vi "Select Global Control.vi"(6 "Variant in":variant, 7 "Shift Pressed?":bool, 8 "error in (no error)":errorcluster, 10 "QD Combo Box Ref":refnum<vi>, 11 "QD Launch VI Ref":refnum<vi>) -> (0 "error out":errorcluster, 4 "Variant out":variant)   [LabVIEW 2017]
doc: "This plugin automatically changes the selected global's selected control. To use it, select the global you want to change, open quickdrop (Ctrl+Space), type the name of the control you want to select from the global, then use this plugin (by default, Ctrl+G).\n\nThe name is case sensitive. If the text in quickdrop does not match any of the controls in the global, or if no global is selected, this plugin does nothing.\n\nDefault Shortcut - [G]"
uses:
  <vilib>/ErrorRing/Error Ring.xnode
panel:
  in  "Undo Name":string="Quick Drop Keyboard Shortcut"
  # "Do not change the connector pane of this VI.\n\nSee the block diagram for directions on how to use this template."
  # "Specify the name of the Undo transaction"
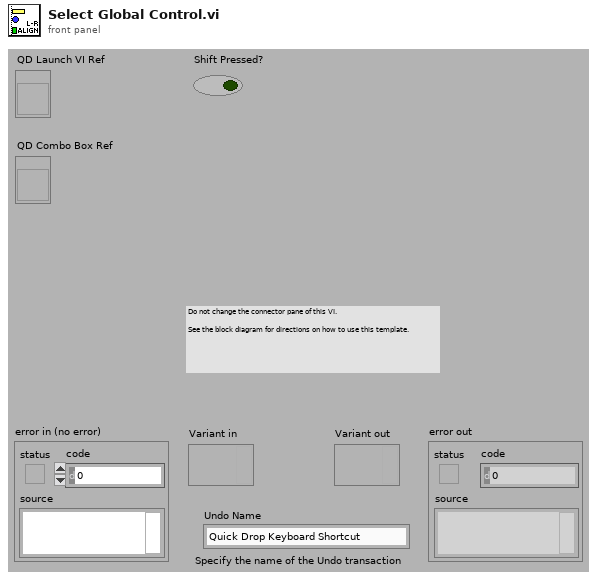
[diagram p1: front panel]
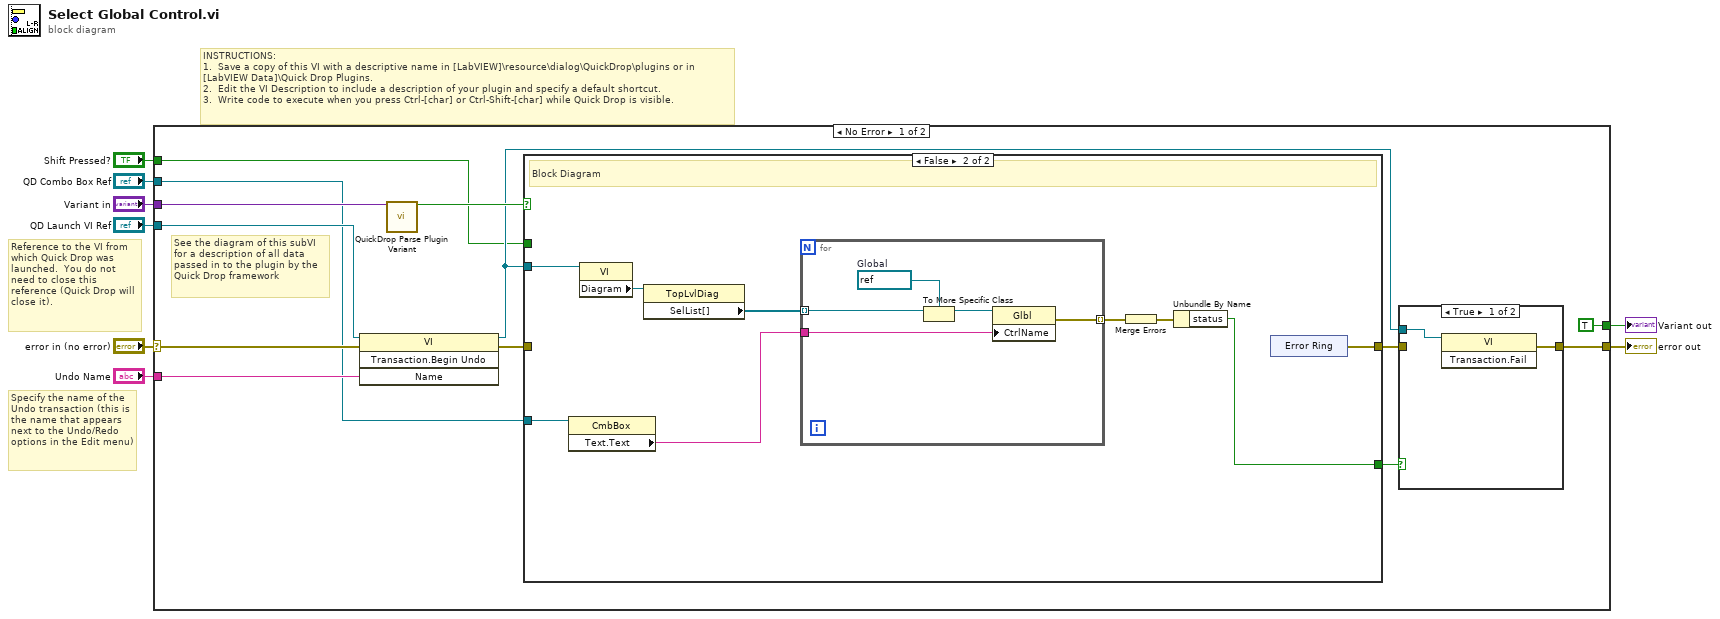
[diagram p0: block diagram]
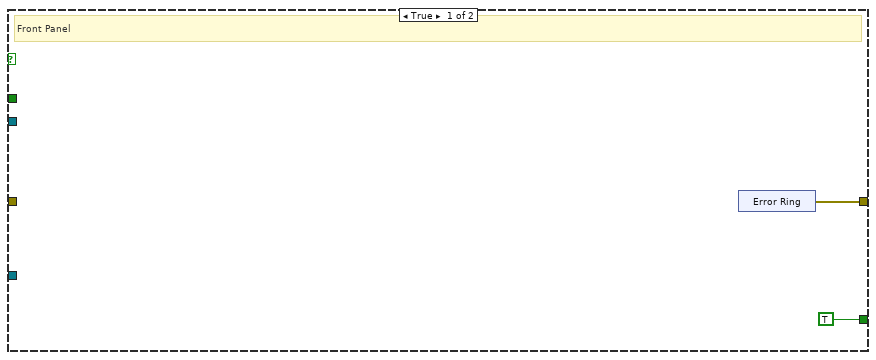
[diagram p2: hidden frame]
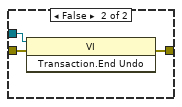
[diagram p3: hidden frame]
diagram:
  # "Specify the name of the Undo transaction (this is the name that appears next to the Undo/Redo options in the Edit menu)"
  # "Reference to the VI from which Quick Drop was launched.  You do not need to close this reference (Quick Drop will close it)."
  # "INSTRUCTIONS:\n1.  Save a copy of this VI with a descriptive name in [LabVIEW]\\resource\\dialog\\QuickDrop\\plugins or in [LabVIEW Data]\\Quick Drop Plugins.\n2.  Edit the VI Description to include a description of your plugin and specify a default shortcut. \n3.  Write code to execute when you press Ctrl-[char] or Ctrl-Shift-[char] while Quick Drop is visible."
  n1 = case shown="No Error" "error in (no error)" {
    selector: "error in (no error)" -> [w20 w45]
    tunnel: [w15 w45] -> w7
    tunnel: "QD Launch VI Ref" -> [w19 _]
    tunnel: "Shift Pressed?" -> [w12 _]
    tunnel: "QD Combo Box Ref" -> [w9 _]
    tunnel: "Variant in" -> [w21 _]
    tunnel: "Undo Name" -> [w18 _]
    tunnel: [TRUE _] -> w1
    frame No Error {
      # "See the diagram of this subVI for a description of all data passed in to the plugin by the Quick Drop framework"
      n2 = invoke class="VI" method="Transaction.Begin Undo"(reference=w19, error in=w20, "Name"=w18) -> (reference out=w14:refnum<vi>, error out=w13:errorcluster)  [unwired: 1 in, 2 out]
      n3 = call <vilib>:"QuickDrop Parse Plugin Variant.vi"("QDKS Variant in"=w21) -> ("QD Launch VI Panel?"=w16:bool)  [unwired: 12 in, 2 out]
      n4 = case shown="False" w16 {
        tunnel: w13 -> [_ _]
        tunnel: w14 -> [_ w32]
        tunnel: w12 -> [_ _]
        tunnel: [w23 w33] -> w11
        tunnel: [TRUE w27] -> w10
        tunnel: w9 -> [_ w29]
        frame True {
          # "Front Panel"
          n5 = xnode "Error Ring"() -> ("error out"=w23:errorcluster)
        }
        frame False {
          # "Block Diagram"
          n6 = property class="CmbBox"(reference=w29) -> ("Text.Text"=w28:string)  [unwired: 1 in, 2 out]
          n7 = property class="VI"(reference=w32) -> ("Diagram"=w31:refnum<vi>)  [unwired: 1 in, 2 out]
          n8 = property class="TopLvlDiag"(reference=w31) -> ("SelList[]"=w30:refnum<vi>[])  [unwired: 1 in, 2 out]
          n9 = for {
            tunnel: w30 -> [w38] mode=indexing
            tunnel: [w35] -> w26 mode=indexing
            tunnel: w28 -> [w34]
            w37 = refnum<vi> refnum  # Global
            n10 = To More Specific Class(target class=w37, reference=w38) -> (specific class reference=w36:refnum<vi>)  [unwired: 1 in, 1 out]
            n11 = property class="Glbl"(reference=w36, "CtrlName"=w34) -> (error out=w35:errorcluster)  [unwired: 1 in, 1 out]
          }
          n12 = Merge Errors(w26) -> (w25:errorcluster)
          n13 = Unbundle By Name(w25) -> ("status"=w27:bool)
          n14 = xnode "Error Ring"() -> ("error out"=w33:errorcluster)
        }
      }
      n15 = case shown="True" w10 {
        tunnel: w14 -> [w40 w43]
        tunnel: [w41 w44] -> w15
        tunnel: w11 -> [_ w42]
        frame True {
          n16 = invoke class="VI" method="Transaction.Fail"(reference=w40) -> (error out=w41:errorcluster)  [unwired: 2 in, 2 out]
        }
        frame False {
          n17 = invoke class="VI" method="Transaction.End Undo"(reference=w43, error in=w42) -> (error out=w44:errorcluster)  [unwired: 1 in, 2 out]
        }
      }
    }
    frame Error {
    }
  }
  "error out" <- w7
  "Variant out" <- w1
